vi "Auto Drive Controls.vi"(0 "X axis value":dbl, 1 "Y axis value":dbl, 2 "Intake Up":bool=TRUE, 3 "Tomahawk Up":bool=TRUE, 4 "Shift High":bool) -> ()   [LabVIEW 2015]
uses:
  <vilib>/Rock Robotics/WPI/Utilities/WPI_GetSetVariantRefNum.vi
  <vilib>/Rock Robotics/WPI/Solenoid/Deprecated/WPI_SolenoidSetBool.vi
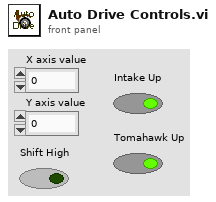
[diagram p1: front panel]
types:
  T1 = typedef "WPI_RobotDriveDevRef.ctl" = cluster{"DevStatus":errorcluster, "Motors[]":T2[], "Square Inputs":bool, "Max Output":dbl}
  T2 = typedef "WPI_MotorControlDeviceRef.ctl" = cluster{"DeviceStatus":errorcluster, "Type":T3, "PWM":cluster{"PWM Channel":T4, "DeadBand":T5}, "CAN":cluster{"Device Number":u8, "Control Mode":T6, "Semaphore":T7, "Max Vout":dbl, "TalonSRX Control Mode":T8}, "Invert":bool}
  T3 = typedef "WPI_MotorControlType.ctl" = enum16{"PWM", "CAN", "CANTalonSRX"}
  T4 = typedef "FPGA_DIOPWMChannel.ctl" = enum8{"PWM 0", "PWM 1", "PWM 2", "PWM 3", "PWM 4", "PWM 5", "PWM 6", "PWM 7", "PWM 8", "PWM 9", "PWM MXP 0", "PWM MXP 1", "PWM MXP 2", "PWM MXP 3", "PWM MXP 4", "PWM MXP 5", "PWM MXP 6", "PWM MXP 7", "PWM MXP 8", "PWM MXP 9", "Invalid"}
  T5 = typedef "WPI_PWMDeadband.ctl" = cluster{"Name":string, "maxPositivePwm":i32, "minPositivePwm":i32, "centerPwm":i32, "maxNegativePwm":i32, "minNegativePwm":i32, "angularRange":u16}
  T6 = typedef "WPI_CANJaguar_ControlMode.ctl" = enum8{"Percent VBus", "Current", "Speed", "Position", "Voltage"}
  T7 = typedef "Semaphore RefNum" = refnum<k1>
  T8 = typedef "WPI_CANTalonSRX_APIControlMode.ctl" = enum8{"Percent VBus", "Speed", "Position", "Slave", "Unchanged / Invalid", "Voltage Compensation", "Current", "Motion Profile"}
  T9 = typedef "WPI_SolenoidDevRef.ctl" = cluster{"DevStatus":errorcluster, "Pneumatics Control Module":u8, "Forward Solenoid Channel":T10, "Reverse Solenoid Channel":T10}
  T10 = typedef "WPI_SolenoidChannel.ctl" = enum8{"Solenoid 0", "Solenoid 1", "Solenoid 2", "Solenoid 3", "Solenoid 4", "Solenoid 5", "Solenoid 6", "Solenoid 7", "Invalid"}
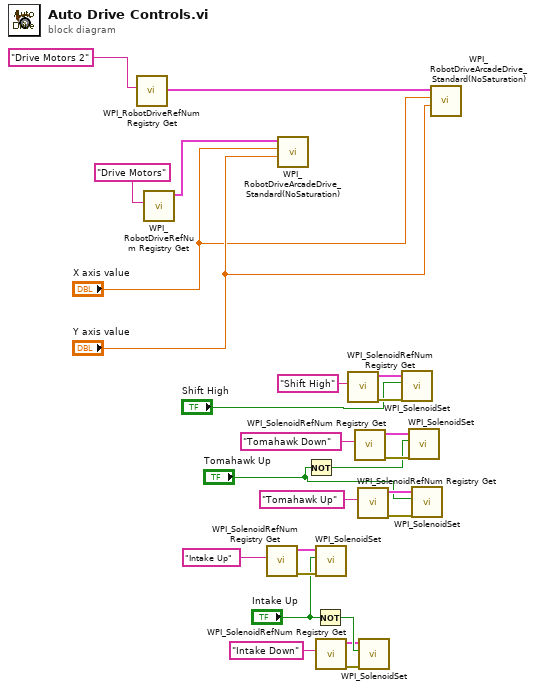
[diagram p0: block diagram]
diagram:
  n1 = call <vilib>:"WPI_RobotDriveRefNum Registry Get.vi"("refnum name"="Drive Motors 2") -> ("RobotDriveDevRef"=w25:T1)  [unwired: 1 in, 9 out]
  n2 = call <vilib>:"WPI_RobotDriveRefNum Registry Get.vi"("refnum name"="Drive Motors") -> ("RobotDriveDevRef"=w23:T1)  [unwired: 1 in, 9 out]
  n3 = call <vilib>:"WPI_SolenoidRefNum Registry Get.vi"("refnum name"="Intake Up") -> ("error out"=w8:errorcluster, "SolenoidDevRef"=w9:T9)  [unwired: 9 in]
  n4 = call <vilib>:"WPI_RobotDriveArcadeDrive_Standard(NoSaturation).vi"("Y axis value"="Y axis value", "X axis value"="X axis value", "RobotDriveDevRef"=w23) -> ()  [unwired: 1 in, 8 out]
  n5 = Not(x="Tomahawk Up") -> (.not. x?=w6:bool)
  n6 = Not(x="Intake Up") -> (.not. x?=w5:bool)
  n7 = call-poly <vilib>:"WPI_SolenoidSet.vi"("error in (no error)"=w8, "Value"="Intake Up", "SolenoidDevRef"=w9) -> ()  [unwired: 7 in, 2 out]
  n8 = call <vilib>:"WPI_SolenoidRefNum Registry Get.vi"("refnum name"="Intake Down") -> ("error out"=w12:errorcluster, "SolenoidDevRef"=w1:T9)  [unwired: 9 in]
  n9 = call <vilib>:"WPI_SolenoidRefNum Registry Get.vi"("refnum name"="Shift High") -> ("error out"=w20:errorcluster, "SolenoidDevRef"=w19:T9)  [unwired: 9 in]
  n10 = call <vilib>:"WPI_SolenoidRefNum Registry Get.vi"("refnum name"="Tomahawk Down") -> ("error out"=w13:errorcluster, "SolenoidDevRef"=w2:T9)  [unwired: 9 in]
  n11 = call <vilib>:"WPI_SolenoidRefNum Registry Get.vi"("refnum name"="Tomahawk Up") -> ("error out"=w17:errorcluster, "SolenoidDevRef"=w16:T9)  [unwired: 9 in]
  n12 = call-poly <vilib>:"WPI_SolenoidSet.vi"("error in (no error)"=w12, "Value"=w5, "SolenoidDevRef"=w1) -> ()  [unwired: 7 in, 2 out]
  n13 = call-poly <vilib>:"WPI_SolenoidSet.vi"("error in (no error)"=w20, "Value"="Shift High", "SolenoidDevRef"=w19) -> ()  [unwired: 7 in, 2 out]
  n14 = call-poly <vilib>:"WPI_SolenoidSet.vi"("error in (no error)"=w13, "Value"=w6, "SolenoidDevRef"=w2) -> ()  [unwired: 7 in, 2 out]
  n15 = call-poly <vilib>:"WPI_SolenoidSet.vi"("error in (no error)"=w17, "Value"="Tomahawk Up", "SolenoidDevRef"=w16) -> ()  [unwired: 7 in, 2 out]
  n16 = call <vilib>:"WPI_RobotDriveArcadeDrive_Standard(NoSaturation).vi"("Y axis value"="Y axis value", "X axis value"="X axis value", "RobotDriveDevRef"=w25) -> ()  [unwired: 1 in, 8 out]
